vi "Init.vi"(8 "error in (no error)":errorcluster, 11 "PSU in":refnum<class "PSU.lvclass">) -> (0 "error out":errorcluster, 3 "PSU out":refnum<class "PSU.lvclass">)   [LabVIEW 2020, in "High Level PSU With Tests.lvlib" / "PSU.lvclass"]
uses:
  PSU.lvclass
  PSU.lvclass/PSU.ctl
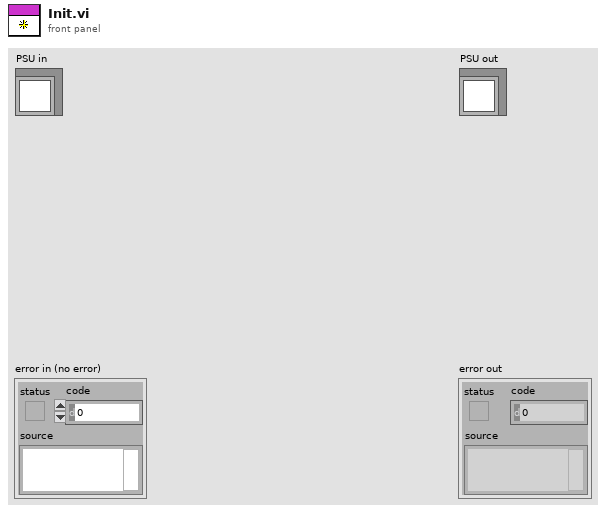
[diagram p1: front panel]
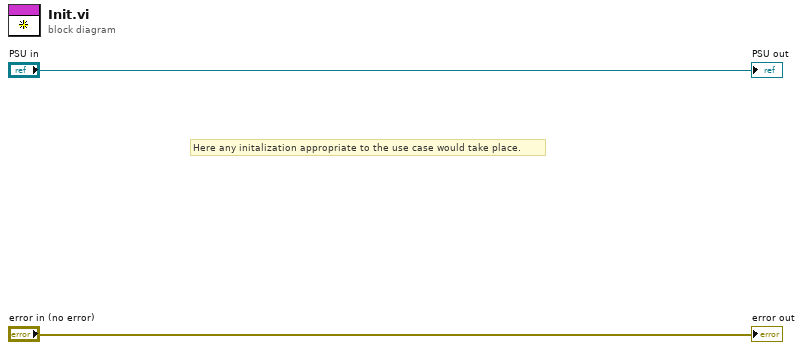
[diagram p0: block diagram]
diagram:
  # "Here any initalization appropriate to the use case would take place."
  "error out" <- "error in (no error)"
  "PSU out" <- "PSU in"
